vi "Slave Stop.vi"(8 "error in (no error)":errorcluster, 9 "ID":i32, 11 "Master in":refnum<class "Master.lvclass">) -> (0 "error out":errorcluster, 3 "Master out":refnum<class "Master.lvclass">)   [LabVIEW 2021, in "Master.lvlib" / "Master.lvclass"]
uses:
  Master.lvclass
  Master.lvclass/Master.ctl
  85d5377b-a5f5-44e6-9c4d-1432076714f8.vi
  <vilib>/Comparison/Equal/Equal Functor/Equal Functor.lvclass
  Slave/Slave.lvlib
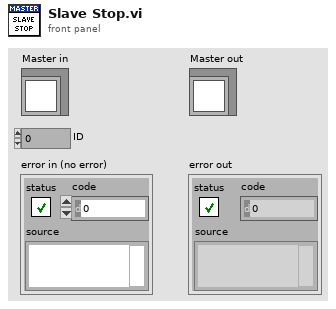
[diagram p1: front panel]
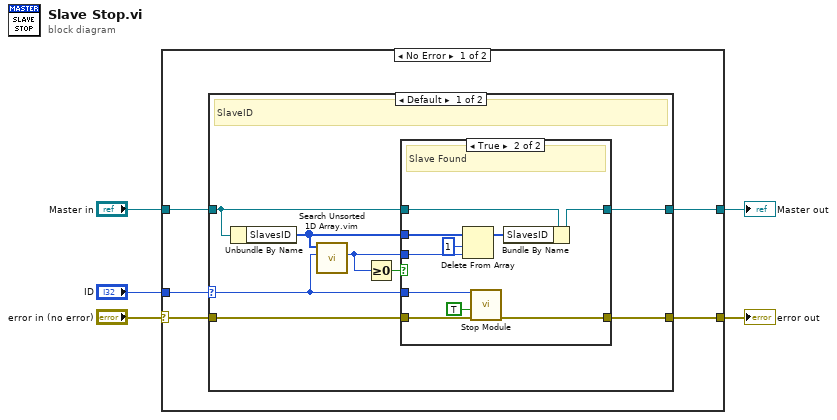
[diagram p0: block diagram]
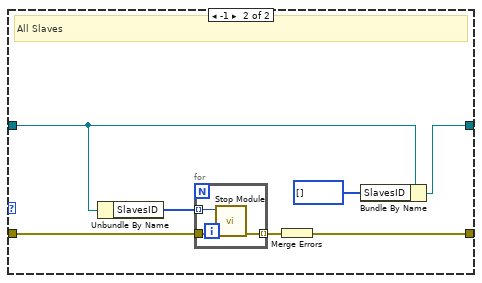
[diagram p3: hidden frame]
diagram:
  n1 = case shown="No Error" "error in (no error)" {
    selector: "error in (no error)" -> [w8 w42]
    tunnel: [w7 w42] -> w4
    tunnel: [w9 w41] -> w2
    tunnel: "Master in" -> [w10 w41]
    tunnel: "ID" -> [w6 _]
    frame No Error {
      n2 = case shown="Default" w6 {
        selector: w6 -> [w11 _]
        tunnel: w8 -> [w18 w37]
        tunnel: [w17 w32] -> w7
        tunnel: w10 -> [w15 w35]
        tunnel: [w14 w34] -> w9
        frame Default {
          # "SlaveID"
          n3 = Unbundle By Name(w15) -> ("SlavesID"=w13:i32[])
          n4 = call "Search Unsorted 1D Array.vim"("element"=w11, "unsorted 1D array"=w13) -> ("index of element"=w12:i32)  [unwired: 9 in]
          n5 = Greater Or Equal To 0?(x=w12) -> (x >= 0?=w16:bool)
          n6 = case shown="True" w16 {
            tunnel: w18 -> [w20 w30]
            tunnel: [w20 w29] -> w17
            tunnel: w11 -> [_ w28]
            tunnel: w15 -> [w19 w27]
            tunnel: [w19 w26] -> w14
            tunnel: w13 -> [_ w24]
            tunnel: w12 -> [_ w22]
            frame False {
              # "Slave Not Found"
            }
            frame True {
              # "Slave Found"
              n7 = Delete From Array(array=w24, length=1, index=w22) -> (array with subset deleted=w25:i32[])  [unwired: 1 out]
              n8 = call "Stop Module.vi"("error in"=w30, "Wait for Module to stop? (F)"=TRUE, "Module ID"=w28) -> ("error out"=w29:errorcluster)  [unwired: 8 in]
              n9 = Bundle By Name(cluster=w27, "SlavesID"=w25) -> (w26:refnum<class "Master.lvclass">)
            }
          }
        }
        frame -1 {
          # "All Slaves"
          n10 = Unbundle By Name(w35) -> ("SlavesID"=w33:i32[])
          n11 = for {
            tunnel: w33 -> [w38] mode=indexing
            tunnel: w37 -> [w40]
            tunnel: [w39] -> w36 mode=indexing
            n12 = call "Stop Module.vi"("error in"=w40, "Module ID"=w38) -> ("error out"=w39:errorcluster)  [unwired: 9 in]
          }
          n13 = Merge Errors(w36) -> (w32:errorcluster)
          n14 = Bundle By Name(cluster=w35, "SlavesID"=i32[] [] ("ClonesID")) -> (w34:refnum<class "Master.lvclass">)
        }
      }
    }
    frame Error {
    }
  }
  "error out" <- w4
  "Master out" <- w2
